vi "dvp Vi Get Saturation State.vi"(10 "pSaturationState":i32, 11 "handle":u32) -> (2 "pSaturationState out":i32, 3 "function return":u32(ring))   [LabVIEW 2018, in "LabViewDVPCamera.lvlib"]
doc: "LabviewDvp2Api dvpStatus dvpViGetSaturationState(dvpHandle handle, BOOL *pSaturationState);"
uses:
  LabViewDVPCamera.lvlib
  LabViewDVPCamera/LabViewDVPCamera.dll
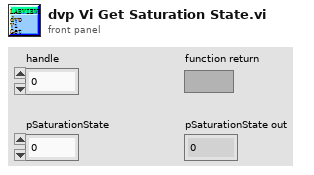
[diagram p1: front panel]
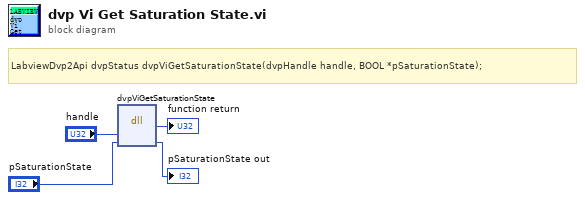
[diagram p0: block diagram]
diagram:
  # "LabviewDvp2Api dvpStatus dvpViGetSaturationState(dvpHandle handle, BOOL *pSaturationState);"
  n1 = dll-call lib="C:/Program Files (x86)/DVP2 Labview cn 64/Sample/LabViewDVPCamera/LabViewDVPCamera.*" fn="dvpViGetSaturationState"("handle"="handle", "pSaturationState"="pSaturationState") -> (→"function return":u32, "pSaturationState"=→"pSaturationState out":i32)  [unwired: 4 in, 2 out]
